vi "DCS_raw_to_volts.vi"(9 "DAQ bit size (16)":u16=16, 10 "Max Voltage Amplitude (2.5 V)":dbl=2.5, 11 "Raw Data":dbl[][](array[numeric])) -> (3 "Voltage Data":dbl[][](array[numeric]))   [LabVIEW 2015]
doc: "Takes raw data and converts to voltage given the DAQ bit resolution and voltage amplitude range."
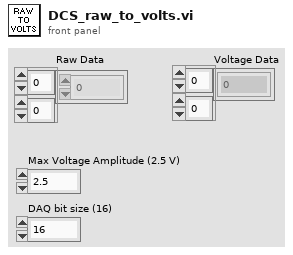
[diagram p1: front panel]
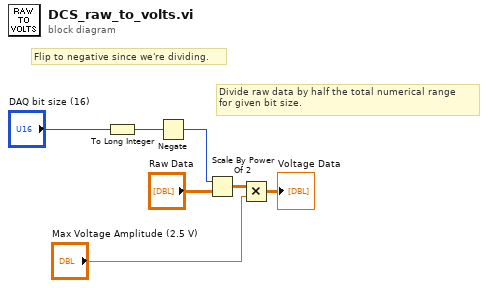
[diagram p0: block diagram]
diagram:
  # "Divide raw data by half the total numerical range \nfor given bit size."
  # "Flip to negative since we're dividing."
  n1 = To Long Integer(number="DAQ bit size (16)") -> (32bit integer=w4:i32)
  n2 = Negate(x=w4) -> (-x=w5:i32)
  n3 = Scale By Power Of 2(n=w5, x="Raw Data") -> (x*2^n=w3:dbl[][])
  n4 = Multiply(x=w3, y="Max Voltage Amplitude (2.5 V)") -> (x*y=→"Voltage Data":dbl[][])
